vi "XIPIN_JESD204_6_2.vi"   [LabVIEW 2017]
doc: "The Xilinx JESD204 core is a fully tested Physical and Data Link Layer block designed to JEDEC JESD204B specifications. An example design and development scripts are provided to facilitate development of a full featured ADC or DAC interface design.\n------------------------------------\n<b>Need License</b> : Yes\n<b>Interface</b> : AXI4 AXI4-Stream"
uses:
  <vilib>/rvi/XilinxIP/XIPIN_XNode/niFpgaXIPIN.xnode
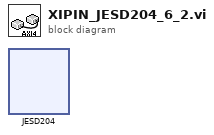
[diagram p0: block diagram]
diagram:
  n1 = xnode ("JESD204")() -> ()
